vi "PicoScope6000Open.vi"(3 "Serial Number":string, 4 "error in (no error)":errorcluster, 5 "Use Serial Number":bool) -> (0 "handle":i16, 1 "Max Adc value":i16, 2 "error out":errorcluster, 6 "Device Info":T1)   [LabVIEW 2020]
doc: "This VI opens a PicoScope 6000 and returns a handle to the device."
uses:
  ps6000.dll
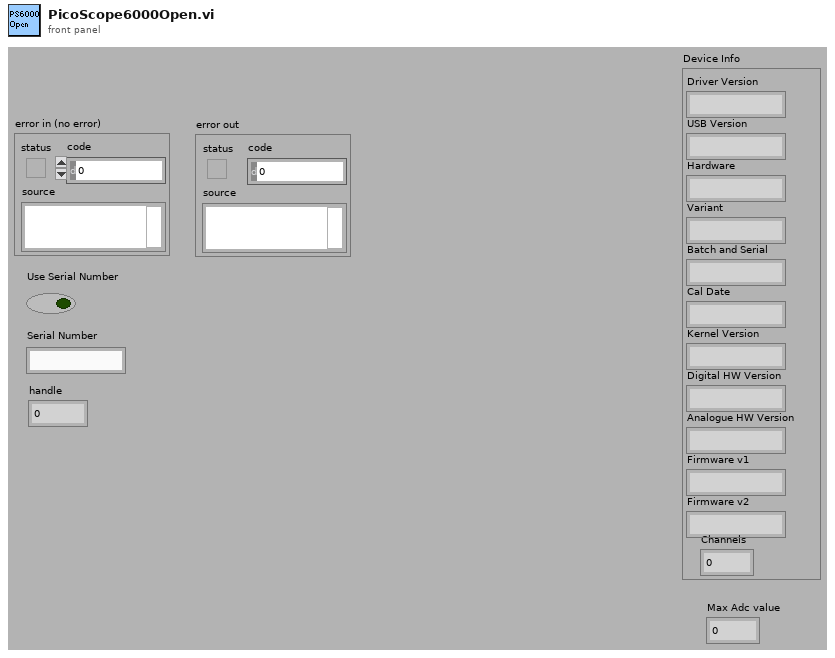
[diagram p1: front panel]
types:
  T1 = cluster{"Driver Version":string, "USB Version":string, "Hardware":string, "Variant":string, "Batch and Serial":string, "Cal Date":string, "Kernel Version":string, "Digital HW Version":string, "Analogue HW Version":string, "Firmware v1":string, "Firmware v2":string, "Channels":i16}
  T2 = cluster{"Driver Version":string, "USB Version":string, "Hardware":string, "Variant":string, "Batch and Serial":string, "Cal Date":string, "Kernel Version":string, "Digital HW Version":string, "Analogue HW Version":string, "Firmware v1":string, "Firmware v2":string}
  T3 = cluster{"Driver Version":string, "USB Version":string, "Hardware":string, "Variant":string, "Batch and Serial":string, "Cal Date":string, "Kernel Version":string, "Digital HW Version":string, "Analogue HW Version":string, "Firmware v1":string, "Firmware v2":string, i16}
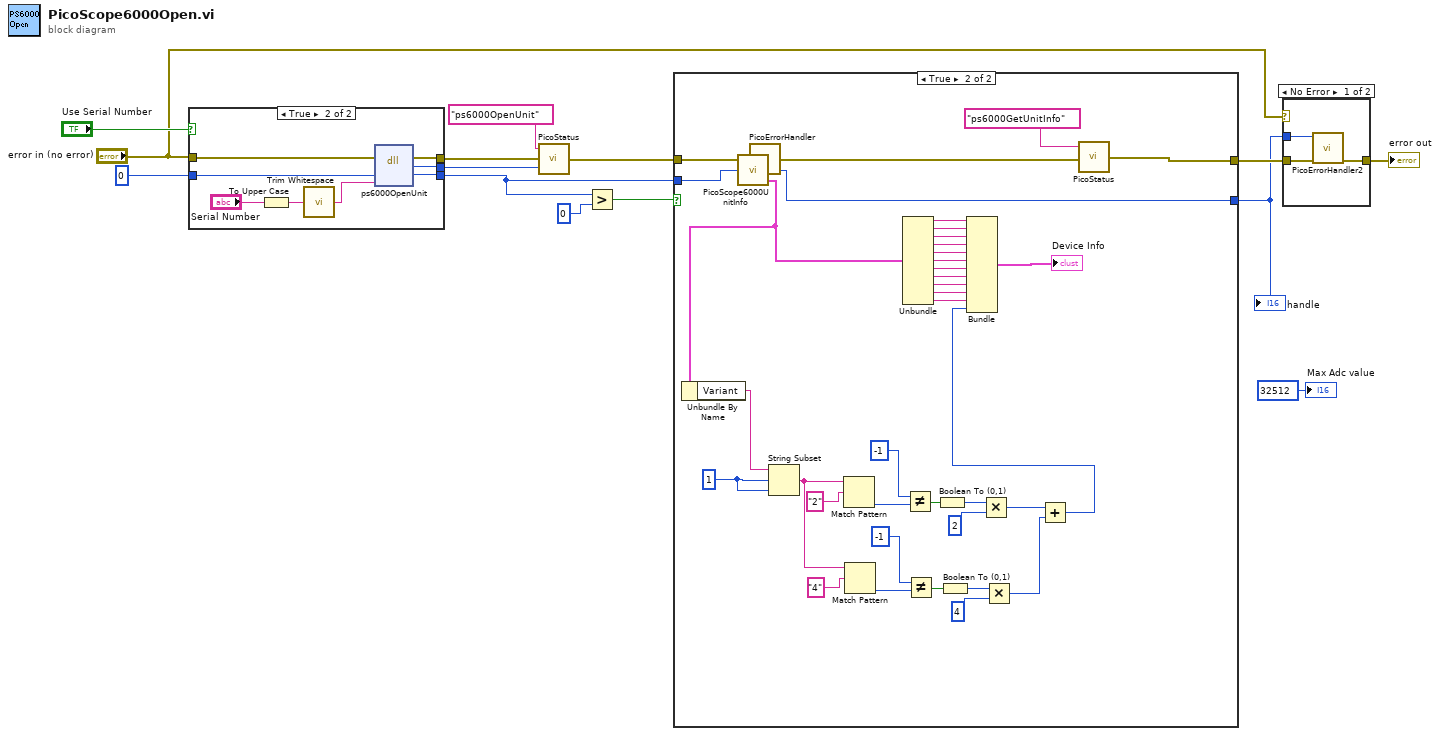
[diagram p0: block diagram]
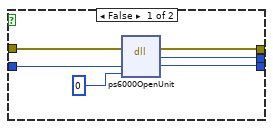
[diagram p4: hidden frame]
diagram:
  n1 = case shown="True" "Use Serial Number" {
    tunnel: "error in (no error)" -> [w20 w24]
    tunnel: i16 0 ("handle") -> [w19 w25]
    tunnel: [w18 w28] -> w11
    tunnel: [w17 w27] -> w10
    tunnel: [w16 w26] -> w6
    frame False {
      n2 = dll-call lib="PS6000.dll" fn="ps6000OpenUnit" ("ps3000.dll:_ps3000_open_unit@0")(error in=w20, "handle"=w19, "serial"=i8 0) -> (error out=w18:errorcluster, "PICO_STATUS"=w17:u32, "handle"=w16:i16)  [unwired: 3 in, 1 out]
    }
    frame True {
      n3 = To Upper Case(1:"Serial Number") -> (0:w22:string)
      n4 = call <vilib>:"Trim Whitespace.vi"("string"=w22) -> ("trimmed string"=w21:string)  [unwired: 1 in]
      n5 = dll-call lib="PS6000.dll" fn="ps6000OpenUnit" ("ps3000.dll:_ps3000_open_unit@0")(error in=w24, "handle"=w25, "serial"=w21) -> (error out=w28:errorcluster, "PICO_STATUS"=w27:u32, "handle"=w26:i16)  [unwired: 3 in, 1 out]
    }
  }
  n6 = call "PicoStatus.vi"("PICO STATUS"=w10, "error in"=w11, "source"="ps6000OpenUnit") -> ("error out"=w8:errorcluster)
  n7 = Greater?(x=w6, y=0) -> (0:w7:bool)
  n8 = case shown="True" w7 {
    tunnel: w6 -> [w29 w67]
    tunnel: w8 -> [w30 w66]
    tunnel: [w30 w64] -> w5
    tunnel: [w29 w62] -> w1
    frame False {
    }
    frame True {
      w49 = 1 ("offset (0)")
      n9 = call "PicoScope6000UnitInfo.vi"("handle in"=w67, "error in (no error)"=w66) -> ("Unit Info"=w61:T2, "handle out"=w62:i16, "error out"=w65:errorcluster)  [unwired: 1 in]
      n10 = Unbundle By Name(w61) -> ("Variant"=w33:string)
      n11 = String Subset(string=w33, offset (0)=w49, length (rest)=w49) -> (substring=w42:string)
      n12 = Match Pattern(string=w42, regular expression="2") -> (offset past match=w47:i32)  [unwired: 1 in, 3 out]
      n13 = Match Pattern(string=w42, regular expression="4") -> (offset past match=w44:i32)  [unwired: 1 in, 3 out]
      n14 = Unbundle(w61) -> ("Driver Version"=w60:string, "USB Version"=w59:string, "Hardware"=w58:string, "Variant"=w57:string, "Batch and Serial"=w56:string, "Cal Date"=w55:string, "Kernel Version"=w54:string, "Digital HW Version"=w53:string, "Analogue HW Version"=w52:string, "Firmware v1"=w51:string, "Firmware v2"=w50:string)
      n15 = Not Equal?(x=-1, y=w47) -> (x != y?=w39:bool)
      n16 = Not Equal?(x=-1, y=w44) -> (x != y?=w35:bool)
      n17 = Boolean To (0,1)(Boolean=w39) -> (0, 1=w38:i16)
      n18 = Boolean To (0,1)(Boolean=w35) -> (0, 1=w36:i16)
      n19 = Multiply(x=w38, y=i16 2) -> (x*y=w41:i16)
      n20 = Multiply(x=w36, y=i16 4) -> (x*y=w34:i16)
      n21 = Add(x=w41, y=w34) -> (x+y=w32:i16)
      n22 = Bundle("Driver Version"=w60, "USB Version"=w59, "Hardware"=w58, "Variant"=w57, "Batch and Serial"=w56, "Cal Date"=w55, "Kernel Version"=w54, "Digital HW Version"=w53, "Analogue HW Version"=w52, "Firmware v1"=w51, "Firmware v2"=w50, w32) -> (→"Device Info":T3)  [unwired: 1 in]
      n23 = call "PicoStatus.vi"("error in"=w65, "source"="ps6000GetUnitInfo") -> ("error out"=w64:errorcluster)  [unwired: 1 in]
    }
  }
  "handle" <- w1
  n24 = call "PicoErrorHandler.vi"() -> ()  [unwired: 1 in, 1 out]
  n25 = case shown="No Error" "error in (no error)" {
    tunnel: [w70 w71] -> w4
    tunnel: w5 -> [w69 w71]
    tunnel: w1 -> [w68 _]
    frame No Error {
      n26 = call "PicoErrorHandler2.vi"("error in (no error)"=w69, "handle In"=w68) -> ("error out"=w70:errorcluster)  [unwired: 9 in]
    }
    frame Error {
    }
  }
  "error out" <- w4
  "Max Adc value" <- i16 32512 ("Max Adc value")
